vi "systemInfo.vi"(1 "read buffer":string) -> (0 "输出簇":T1)   [LabVIEW 2014]
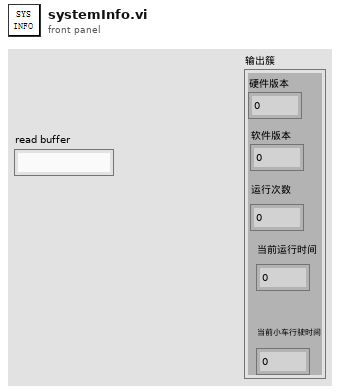
[diagram p1: front panel]
types:
  T1 = cluster{"硬件版本":u16, "软件版本":u16, "运行次数\n":u16, "当前运行时间":u16, "当前小车行驶时间":u16}
  T2 = cluster{"16位整型":u16, "16位整型":u16, "16位整型":u16, "16位整型":u16, "16位整型":u16}
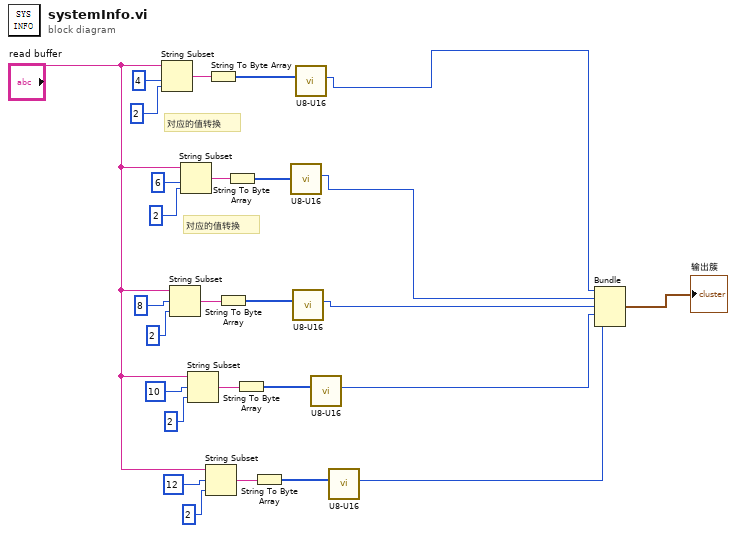
[diagram p0: block diagram]
diagram:
  # "对应的值转换"
  # "对应的值转换"
  n1 = String Subset(string="read buffer", offset (0)=4 ("长度（剩余）"), length (rest)=2 ("长度（剩余）")) -> (substring=w24:string)
  n2 = String Subset(string="read buffer", offset (0)=8 ("长度（剩余）"), length (rest)=2 ("长度（剩余）")) -> (substring=w27:string)
  n3 = String Subset(string="read buffer", offset (0)=6 ("长度（剩余）"), length (rest)=2 ("长度（剩余）")) -> (substring=w19:string)
  n4 = String Subset(string="read buffer", offset (0)=10 ("长度（剩余）"), length (rest)=2 ("长度（剩余）")) -> (substring=w15:string)
  n5 = String Subset(string="read buffer", offset (0)=12 ("长度（剩余）"), length (rest)=2 ("长度（剩余）")) -> (substring=w6:string)
  n6 = String To Byte Array(string=w24) -> (unsigned byte array=w10:u8[])
  n7 = String To Byte Array(string=w27) -> (unsigned byte array=w20:u8[])
  n8 = String To Byte Array(string=w19) -> (unsigned byte array=w9:u8[])
  n9 = String To Byte Array(string=w15) -> (unsigned byte array=w12:u8[])
  n10 = String To Byte Array(string=w6) -> (unsigned byte array=w3:u8[])
  n11 = call "U8-U16.vi"("数组"=w9) -> ("16位整型"=w7:u16)  [unwired: 8 in, 1 out]
  n12 = call "U8-U16.vi"("数组"=w20) -> ("16位整型"=w16:u16)  [unwired: 8 in, 1 out]
  n13 = call "U8-U16.vi"("数组"=w10) -> ("16位整型"=w8:u16)  [unwired: 8 in, 1 out]
  n14 = call "U8-U16.vi"("数组"=w12) -> ("16位整型"=w11:u16)  [unwired: 8 in, 1 out]
  n15 = call "U8-U16.vi"("数组"=w3) -> ("16位整型"=w1:u16)  [unwired: 8 in, 1 out]
  n16 = Bundle("16位整型"=w8, "16位整型"=w7, "16位整型"=w16, "16位整型"=w11, "16位整型"=w1) -> (→"输出簇":T2)  [unwired: 1 in]
